vi "Self Configure.vi"(8 "error in":errorcluster, 11 "Oscilloscope in":refnum<class "Oscilloscope.lvclass">) -> (0 "error out":errorcluster, 3 "Oscilloscope out":refnum<class "Oscilloscope.lvclass">)   [LabVIEW 2019, in "Oscilloscope.lvlib" / "Oscilloscope.lvclass"]
uses:
  Oscilloscope.lvclass
  Oscilloscope.lvclass/Oscilloscope.ctl
  builds/Tools/Config.lvlibp/Config.lvclass
  C:/Users/Public/Documents/Development/builds/Tools/Config.lvlibp/Config.lvclass
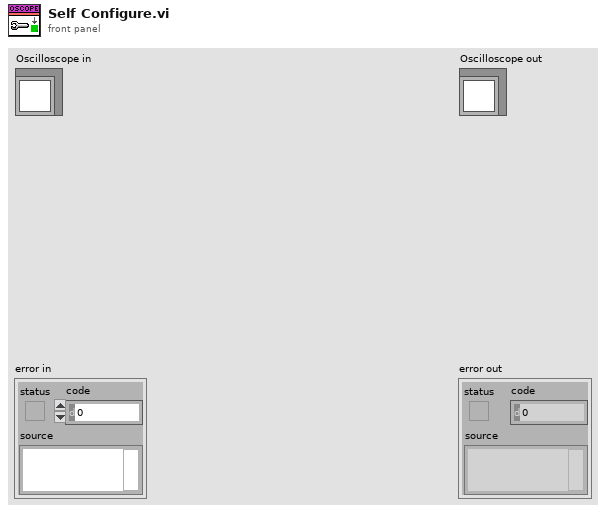
[diagram p1: front panel]
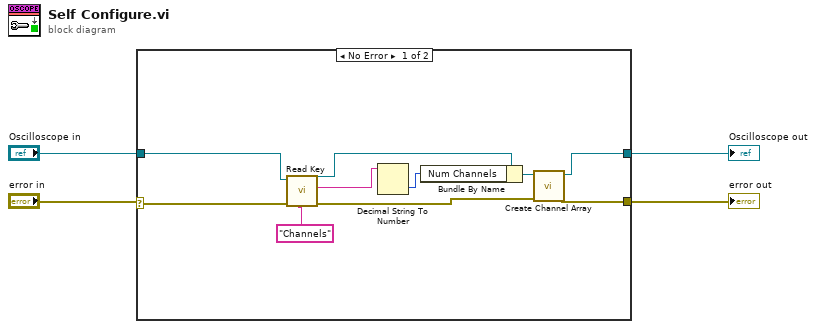
[diagram p0: block diagram]
diagram:
  n1 = case shown="No Error" "error in" {
    selector: "error in" -> [w10 w16]
    tunnel: [w14 w15] -> w4
    tunnel: [w13 w16] -> w3
    tunnel: "Oscilloscope in" -> [w7 w15]
    frame No Error {
      n2 = call "Read Key.vi"("Key Name"="Channels", "error in"=w10, "Config in"=w7) -> ("error out"=w9:errorcluster, "Key Value"=w5:string, "Config out"=w6:refnum<class "Oscilloscope.lvclass">)  [unwired: 6 in]
      n3 = Decimal String To Number(string=w5) -> (number=w11:i32)  [unwired: 2 in, 1 out]
      n4 = Bundle By Name(cluster=w6, "Num Channels"=w11) -> (w12:refnum<class "Oscilloscope.lvclass">)
      n5 = call "Create Channel Array.vi"("error in"=w9, "Oscilloscope in"=w12) -> ("error out"=w13:errorcluster, "Oscilloscope out"=w14:refnum<class "Oscilloscope.lvclass">)  [unwired: 8 in]
    }
    frame Error {
    }
  }
  "error out" <- w3
  "Oscilloscope out" <- w4
